vi "Map_Create.vi"(0 "reference in":refnum<class "Map.lvclass">, 5 "error in (no error)":errorcluster) -> (14 "reference out":refnum<class "Map.lvclass">, 19 "error out":errorcluster)   [LabVIEW 2019, in "Map.lvclass"]
doc: "This VI creates a Map/Maze object"
uses:
  Map.lvclass
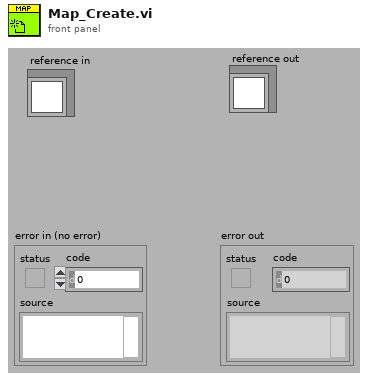
[diagram p1: front panel]
types:
  T1 = typedef "Map.lvclass/ObjectAttributes.ctl" = cluster{"Width":i32, "Height":i32, "Map":bool[][]}
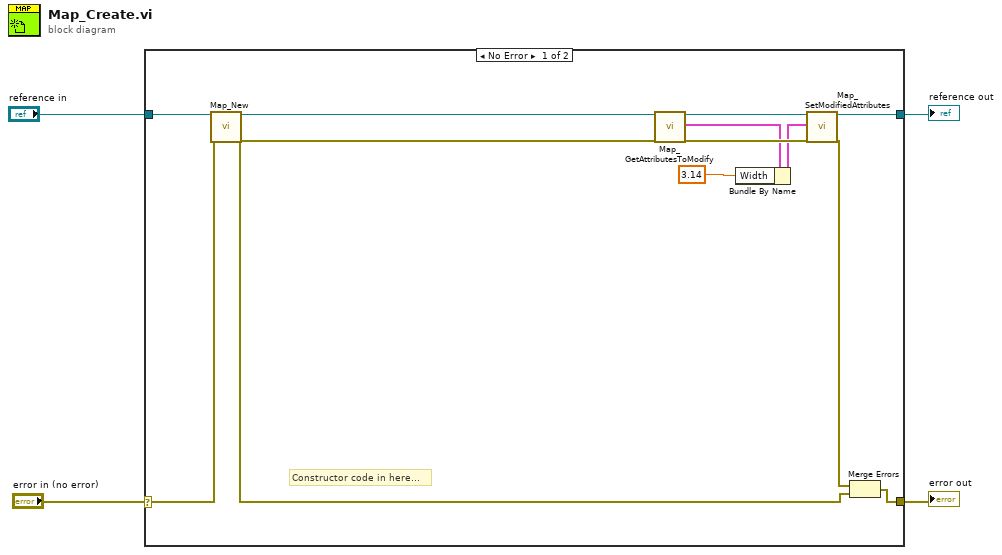
[diagram p0: block diagram]
diagram:
  n1 = case shown="No Error" "error in (no error)" {
    selector: "error in (no error)" -> [w16 w18]
    tunnel: [w7 w18] -> w4
    tunnel: "reference in" -> [w9 w17]
    tunnel: [w10 w17] -> w2
    frame No Error {
      # "Constructor code in here..."
      n2 = call "Map_New.vi"("reference in"=w9, "error in (no error)"=w16) -> ("reference out"=w8:refnum<class "Map.lvclass">, "error out"=w5:errorcluster)  [unwired: 3 in, 13 out]
      n3 = call "Map_GetAttributesToModify.vi"("reference in"=w8, "error in (no error)"=w5) -> ("reference out"=w14:refnum<class "Map.lvclass">, "Attributes"=w13:T1, "error out"=w15:errorcluster)  [unwired: 1 in, 14 out]
      n4 = Bundle By Name(cluster=w13, "Width"=3.14 ("attribute1")) -> (w12:T1)
      n5 = call "Map_SetModifiedAttributes.vi"("reference in"=w14, "Attributes"=w12, "error in (no error)"=w15) -> ("reference out"=w10:refnum<class "Map.lvclass">, "error out"=w6:errorcluster)  [unwired: 3 in, 12 out]
      n6 = Merge Errors(w6, w5) -> (w7:errorcluster)
    }
    frame Error {
    }
  }
  "error out" <- w4
  "reference out" <- w2
